vi "Get Device USB Strings.vi"(8 "error in (no error)":errorcluster, 11 "device index":u32) -> (0 "error out":errorcluster, 1 "Serial Number":string, 2 "Product Name":string, 3 "Manufacturer Name":string)   [LabVIEW 2019, in "RTL-SDR.lvlib"]
uses:
  RTL-SDR.lvlib
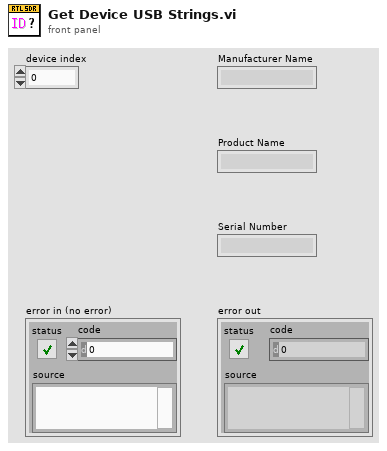
[diagram p1: front panel]
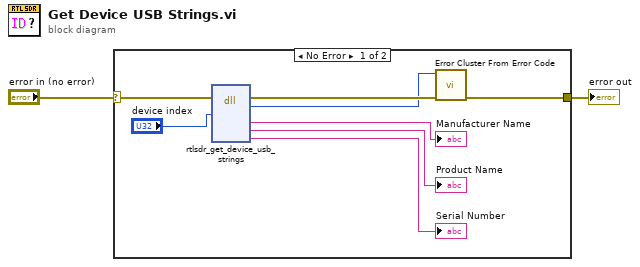
[diagram p0: block diagram]
diagram:
  n1 = case shown="No Error" "error in (no error)" {
    selector: "error in (no error)" -> [w8 w11]
    tunnel: [w9 w11] -> w2
    frame No Error {
      n2 = dll-call lib="usr/local/Cellar/librtlsdr/0.6.0/bin/rtl_sdr" fn="rtlsdr_get_device_usb_strings"(error in=w8, "index"="device index") -> (error out=w10:errorcluster, "return type"=w4:i32, "manufact"=→"Manufacturer Name":string, "product"=→"Product Name":string, "serial"=→"Serial Number":string)  [unwired: 6 in, 1 out]
      n3 = call <vilib>:"Error Cluster From Error Code.vi"("error in (no error)"=w10, "error code (0)"=w4) -> ("error out"=w9:errorcluster)  [unwired: 7 in]
    }
    frame Error {
    }
  }
  "error out" <- w2
